vi "GaGe4_Start.vi"(8 "error in (no error)":errorcluster, 11 "Handle Cluster":T1) -> (0 "error out":errorcluster)   [LabVIEW 2015]
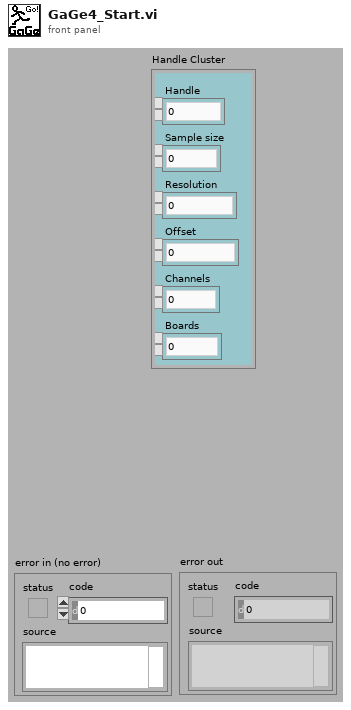
[diagram p1: front panel]
types:
  T1 = cluster{"Handle":u32, "Sample size":u32, "Resolution":i32, "Offset":i32, "Channels":u32, "Boards":u32}
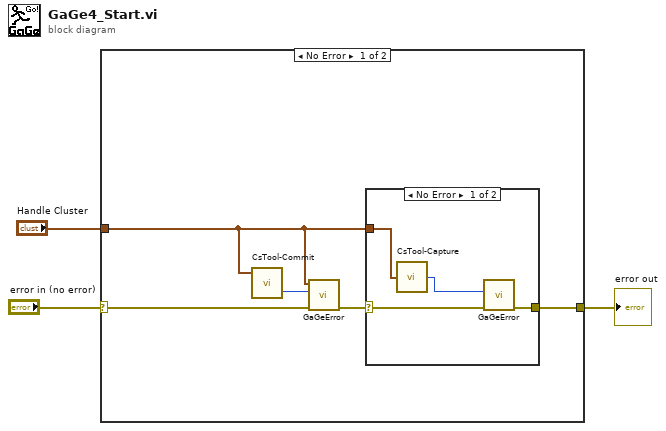
[diagram p0: block diagram]
diagram:
  n1 = case shown="No Error" "error in (no error)" {
    selector: "error in (no error)" -> [w8 w14]
    tunnel: [w5 w14] -> w3
    tunnel: "Handle Cluster" -> [w4 _]
    frame No Error {
      n2 = call "CsTool-Commit.vi"("Handle Cluster"=w4) -> ("Error Code"=w7:i32)  [unwired: 2 in, 1 out]
      n3 = call "GaGeError.vi"("error in (no error)"=w8, "Error Code"=w7, "Handle Cluster"=w4) -> ("error out"=w6:errorcluster)  [unwired: 3 in, 5 out]
      n4 = case shown="No Error" w6 {
        selector: w6 -> [w12 w13]
        tunnel: [w11 w13] -> w5
        tunnel: w4 -> [w10 _]
        frame No Error {
          n5 = call "CsTool-Capture.vi"("Handle Cluster"=w10) -> ("Error Code"=w9:i32)
          n6 = call "GaGeError.vi"("error in (no error)"=w12, "Error Code"=w9) -> ("error out"=w11:errorcluster)  [unwired: 4 in, 5 out]
        }
        frame Error {
        }
      }
    }
    frame Error {
    }
  }
  "error out" <- w3
